vi "Save File Allow Only One Folder Create.vi"(8 "Error In":errorcluster, 10 "Debug or Inv File? in":T2, 11 "LV Program in":T1=enum."DOE Stand") -> (0 "Error Out":errorcluster, 1 "Debug or Inv File? out":T2, 2 "Only One Folder?":bool, 3 "LV Program out":T1)   [LabVIEW 2023, in "Save File.lvlib"]
uses:
  Save File.lvlib
  Private/Type Definitions/Save File Type.ctl
  File Setup (Public)/Type Definition/Save File DOE LabView Program.ctl
  File Setup.lvlib
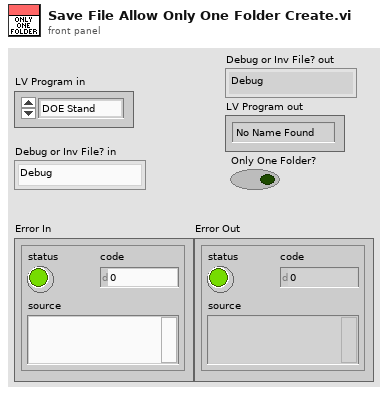
[diagram p1: front panel]
types:
  T1 = typedef "File Setup.lvlib/Save File DOE LabView Program.ctl" = enum16{"No Name Found", "DOE Stand", "Dishwasher Kitchen", "Portable Stand", "HEWH", "Dryer", "Dryer WILT", "HCC", "PRAT", "HEWH RLT", "Refrigeration", "Gas Water Heater"}
  T2 = typedef "Save File Type.ctl" = enum16{"Debug", "Inv and MC", "Current", "Bus File"}
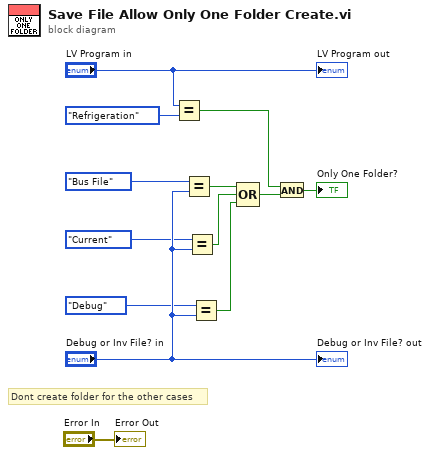
[diagram p0: block diagram]
diagram:
  # "Dont create folder for the other cases"
  n1 = Equal?(x="LV Program in", y=Save_File_DOE_LabView_Program."Refrigeration") -> (x = y?=w11:bool)
  n2 = Equal?(x=Save_File_Type."Bus File", y="Debug or Inv File? in") -> (x = y?=w8:bool)
  n3 = Equal?(x=Save_File_Type."Current", y="Debug or Inv File? in") -> (x = y?=w9:bool)
  n4 = Equal?(x=Save_File_Type."Debug", y="Debug or Inv File? in") -> (x = y?=w10:bool)
  n5 = Compound Arithmetic op=OR(w8, w9, w10) -> (w12:bool)
  n6 = And(x=w11, y=w12) -> (x .and. y?=→"Only One Folder?":bool)
  "Debug or Inv File? out" <- "Debug or Inv File? in"
  "LV Program out" <- "LV Program in"
  "Error Out" <- "Error In"
